vi "Temp_version_creation.vi"() -> ()   [LabVIEW 2014]
panel:
  out "data":string[](array[string])
  out "reversed array":string[](array[string])
  out "channel names":string[](array[string])
  in  "Path":path
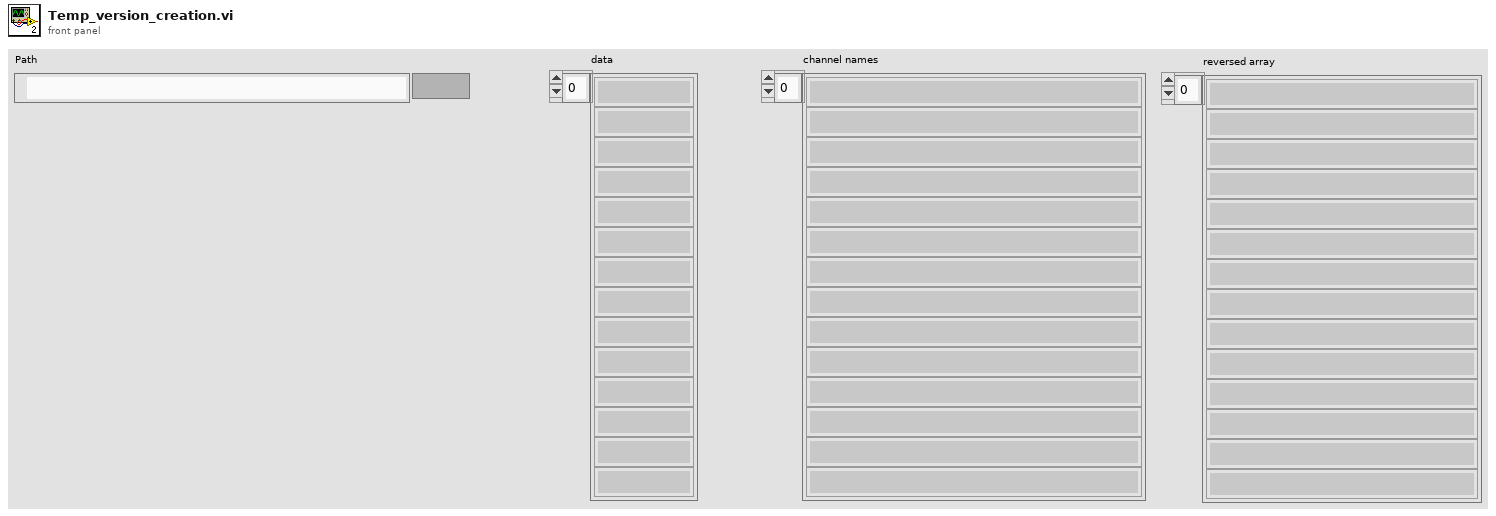
[diagram p1: front panel]
types:
  T1 = enum16{"open", "open or create", "create or replace", "create", "open (read-only)"}
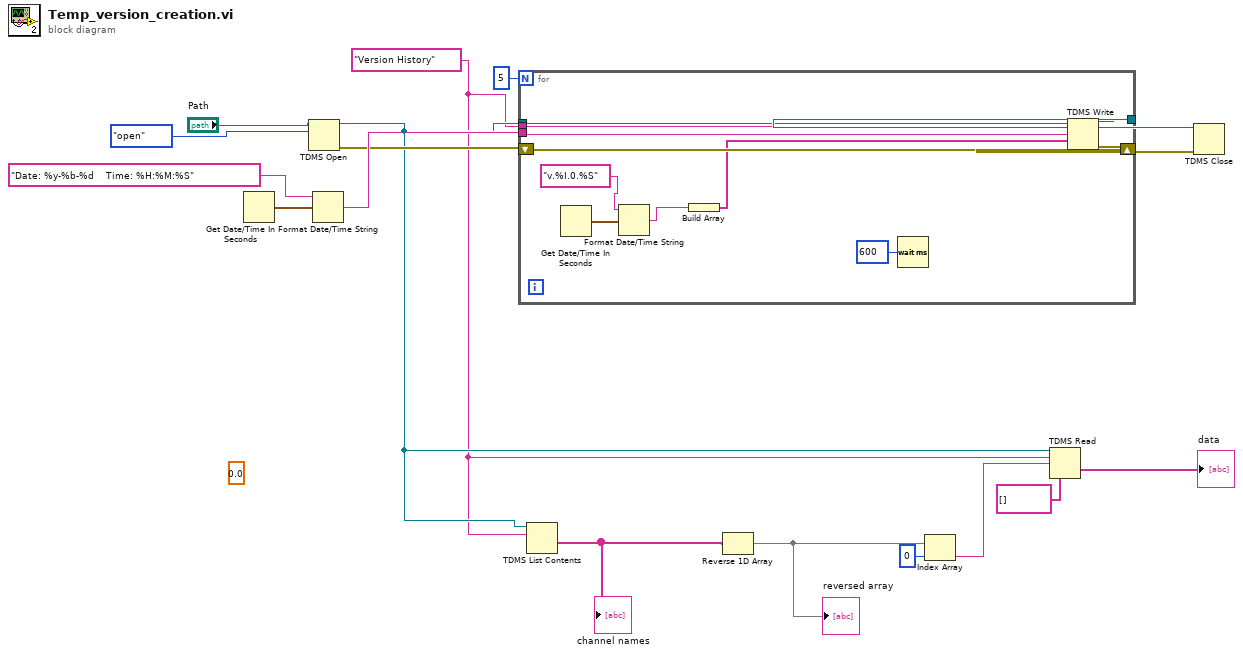
[diagram p0: block diagram]
diagram:
  (unwired) 0.0
  w7 = "Version History" ("group name in (Untitled)")
  n1 = Get Date/Time In Seconds() -> (seconds since 1Jan1904=w15:timestamp)
  n2 = TDMS Open(10:T1."open" ("operation (0:open)"), 11:"Path") -> (0:w10:errorcluster, 3:w8:refnum<k34>)  [unwired: 5 in]
  n3 = Format Date/Time String(time format string (%c)="Date: %y-%b-%d    Time: %H:%M:%S", seconds (now)=w15) -> (date/time string=w13:string)  [unwired: 1 in]
  n4 = for {
    N: 5 -> [_]
    tunnel: w8 -> [w28]
    tunnel: w7 -> [w27]
    tunnel: w13 -> [w22]
    tunnel: [w26] -> w11
    shift-right: [w24] -> w9
    shift-left: w10 -> [w25]
    n5 = Get Date/Time In Seconds() -> (seconds since 1Jan1904=w23:timestamp)
    n6 = Format Date/Time String(time format string (%c)="v.%I.0.%S", seconds (now)=w23) -> (date/time string=w20:string)  [unwired: 1 in]
    n7 = Build Array(w20) -> (w19:string[])
    n8 = Wait (ms)(milliseconds to wait=u32 600) -> ()  [unwired: 1 out]
    n9 = TDMS Write(0:w28, 5:w27, 7:w22, 9:w19, 11:w25) -> (4:w26:refnum<k34>, 15:w24:errorcluster)  [unwired: 1 in, 2 out]
  }
  n10 = TDMS List Contents(6:w7, 7:w8) -> (1:w6:string[])  [unwired: 1 in, 3 out]
  "channel names" <- w6
  n11 = Reverse 1D Array(array=w6) -> (reversed array=w5:string[])
  "reversed array" <- w5
  n12 = Index Array(array=w5, index=0) -> (element=w3:string)
  n13 = TDMS Read(0:w8, 5:w7, 7:w3, 12:string[] []) -> (10:→"data":string[])  [unwired: 4 in, 5 out]
  n14 = TDMS Close(8:w9, 11:w11) -> ()  [unwired: 2 out]
